vi "16-CalculateResult.vi"(10 "Packet in":T1) -> (1 "Result":u64, 2 "Packet out":T1)   [LabVIEW 2019, in "16.lvlib"]
uses:
  16.lvlib
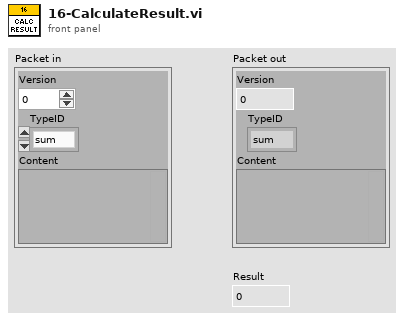
[diagram p1: front panel]
types:
  T1 = cluster{"Version":u32, "TypeID":enum16{"sum", "product", "minimum", "maximum", "literal", "greater than", "less than", "equal to"}, "Content":variant}
  T2 = enum16{"sum", "product", "minimum", "maximum", "literal", "greater than", "less than", "equal to"}
  T3 = cluster{"Version":u32, "TypeID":enum16{"sum", "product", "minimum", "maximum", "literal", "greater than", "less than", "equal to"}, "Content":variant}[]
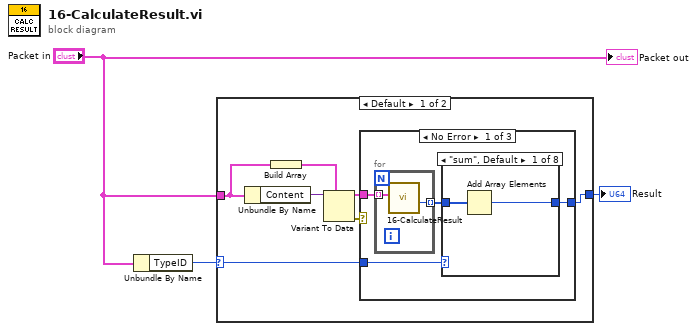
[diagram p0: block diagram]
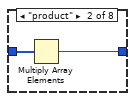
[diagram p2: hidden frame]
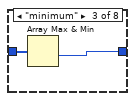
[diagram p3: hidden frame]
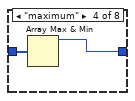
[diagram p4: hidden frame]
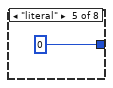
[diagram p5: hidden frame]
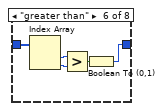
[diagram p6: hidden frame]
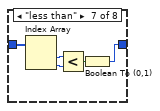
[diagram p7: hidden frame]
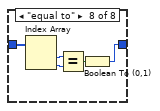
[diagram p8: hidden frame]
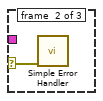
[diagram p9: hidden frame]
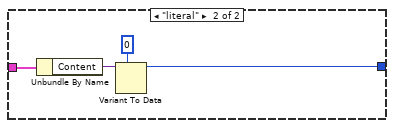
[diagram p11: hidden frame]
diagram:
  n1 = Unbundle By Name("Packet in") -> ("TypeID"=w1:T2)
  n2 = case shown="Default" w1 {
    selector: w1 -> [w7 _]
    tunnel: "Packet in" -> [w9 w45]
    tunnel: [w5 w42] -> w3
    frame Default {
      n3 = Unbundle By Name(w9) -> ("Content"=w10:variant)
      n4 = Build Array(w9) -> (w8:T3)
      n5 = Variant To Data(type=w8, Variant=w10) -> (data=w6:T3, error out=w4:errorcluster)  [unwired: 1 in]
      n6 = case shown="No Error" w4 {
        selector: w4 -> [_ w41 _]
        tunnel: w7 -> [w14 _ _]
        tunnel: w6 -> [w13 _ _]
        tunnel: [w11 _ _] -> w5
        frame #0 {
          n7 = for {
            tunnel: w13 -> [w15] mode=indexing
            tunnel: [w16] -> w12 mode=indexing
            n8 = call "16-CalculateResult.vi"("Packet in"=w15) -> ("Result"=w16:u64)  [unwired: 9 in, 1 out]
          }
          n9 = case shown="\"sum\", Default" w14 {
            tunnel: w12 -> [w18 w20 w22 w24 _ w30 w35 w40]
            tunnel: [w17 w19 w21 w23 u64 0 ("Numeric") w26 w31 w36] -> w11
            frame "sum", Default {
              n10 = Add Array Elements(numeric array=w18) -> (sum=w17:u64)
            }
            frame "product" {
              n11 = Multiply Array Elements(1:w20) -> (0:w19:u64)
            }
            frame "minimum" {
              n12 = Array Max & Min(array=w22) -> (min value=w21:u64)  [unwired: 3 out]
            }
            frame "maximum" {
              n13 = Array Max & Min(array=w24) -> (max value=w23:u64)  [unwired: 3 out]
            }
            frame "literal" {
            }
            frame "greater than" {
              n14 = Index Array(array=w30) -> (element #1=w29:u64, element #2=w28:u64)  [unwired: 2 in]
              n15 = Greater?(x=w29, y=w28) -> (0:w27:bool)
              n16 = Boolean To (0,1)(Boolean=w27) -> (0, 1=w26:i16)
            }
            frame "less than" {
              n17 = Index Array(array=w35) -> (element #1=w34:u64, element #2=w33:u64)  [unwired: 2 in]
              n18 = Less?(x=w34, y=w33) -> (x < y?=w32:bool)
              n19 = Boolean To (0,1)(Boolean=w32) -> (0, 1=w31:i16)
            }
            frame "equal to" {
              n20 = Index Array(array=w40) -> (element #1=w39:u64, element #2=w38:u64)  [unwired: 2 in]
              n21 = Equal?(x=w39, y=w38) -> (x = y?=w37:bool)
              n22 = Boolean To (0,1)(Boolean=w37) -> (0, 1=w36:i16)
            }
          }
        }
        frame #1 {
          n23 = call <vilib>:"Simple Error Handler.vi"("error in (no error)"=w41) -> ()  [unwired: 4 in, 5 out]
        }
        frame #2 {
          # "NULL Packet"
        }
      }
    }
    frame "literal" {
      n24 = Unbundle By Name(w45) -> ("Content"=w44:variant)
      n25 = Variant To Data(type=u64 0, Variant=w44) -> (data=w42:u64)  [unwired: 1 in, 1 out]
    }
  }
  "Result" <- w3
  "Packet out" <- "Packet in"
